vi "Read configuration.vi"(8 "error in (no error)":errorcluster, 11 "DMM in":refnum<class "DMM Instrument.lvclass">) -> (0 "error out":errorcluster, 2 "configuration":refnum<class "CEF_serializable configuration.lvclass">, 3 "DMM out":refnum<class "DMM Instrument.lvclass">)   [LabVIEW 2025, in "DMM.lvlib" / "DMM Instrument.lvclass"]
uses:
  DMM Instrument.lvclass
  Users/Public/Documents/Sandia National Labs/TSS Plugin/CEF.lvlibp/serializable configuration/CEF_serializable configuration.lvclass
  DMM Instrument.lvclass/DMM Instrument.ctl
  DMM configuration/DMM configuration.lvclass
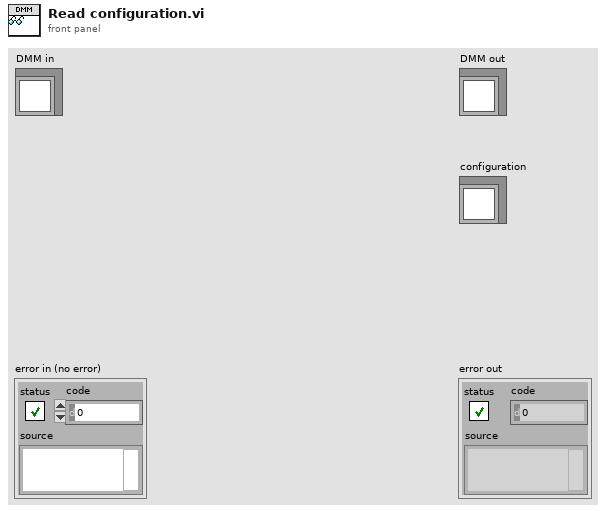
[diagram p1: front panel]
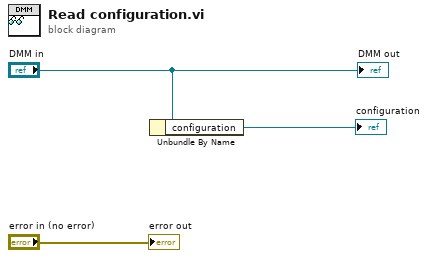
[diagram p0: block diagram]
diagram:
  n1 = Unbundle By Name("DMM in") -> ("configuration"=→"configuration":refnum<class "DMM configuration.lvclass">)
  "error out" <- "error in (no error)"
  "DMM out" <- "DMM in"
